vi "Framework Main.vi"(8 "error in (no error)":errorcluster, 11 "Framework in":refnum<class "Framework.lvclass">) -> (0 "error out":errorcluster, 3 "Framework out":refnum<class "Framework.lvclass">)   [LabVIEW 2017]
uses:
  Builds/Data Sharing Framework/Current/Core/DSF Core.lvlibp/Classes/Framework/Framework.lvclass
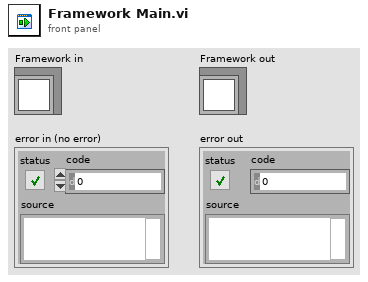
[diagram p1: front panel]
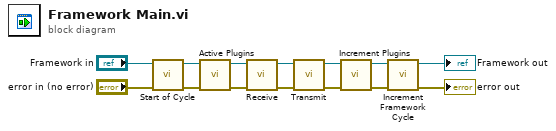
[diagram p0: block diagram]
diagram:
  n1 = call "Start of Cycle.vi"("error in (no error)"="error in (no error)", "Framework in"="Framework in") -> ("error out"=w1:errorcluster, "Framework out"=w2:refnum<class "Framework.lvclass">)  [unwired: 8 in]
  n2 = call "Active Plugins.vi"("error in (no error)"=w1, "Framework in"=w2) -> ("error out"=w5:errorcluster, "Framework out"=w6:refnum<class "Framework.lvclass">)  [unwired: 8 in]
  n3 = call "Receive.vi"("error in (no error)"=w5, "Framework in"=w6) -> ("error out"=w12:errorcluster, "Framework out"=w11:refnum<class "Framework.lvclass">)  [unwired: 8 in]
  n4 = call "Transmit.vi"("error in (no error)"=w12, "Framework in"=w11) -> ("error out"=w13:errorcluster, "Framework out"=w14:refnum<class "Framework.lvclass">)  [unwired: 8 in]
  n5 = call "Increment Plugins.vi"("error in (no error)"=w13, "Framework in"=w14) -> ("error out"=w9:errorcluster, "Framework out"=w10:refnum<class "Framework.lvclass">)  [unwired: 8 in]
  n6 = call "Increment Framework Cycle.vi"("error in (no error)"=w9, "Framework in"=w10) -> ("error out"=→"error out":errorcluster, "Framework out"=→"Framework out":refnum<class "Framework.lvclass">)  [unwired: 8 in]
